vi "SaveScan_IM.vi"(10 "ScanSave Parameter":T1) -> (2 "Result":string)   [LabVIEW 2020]
panel:
  out "error out":errorcluster
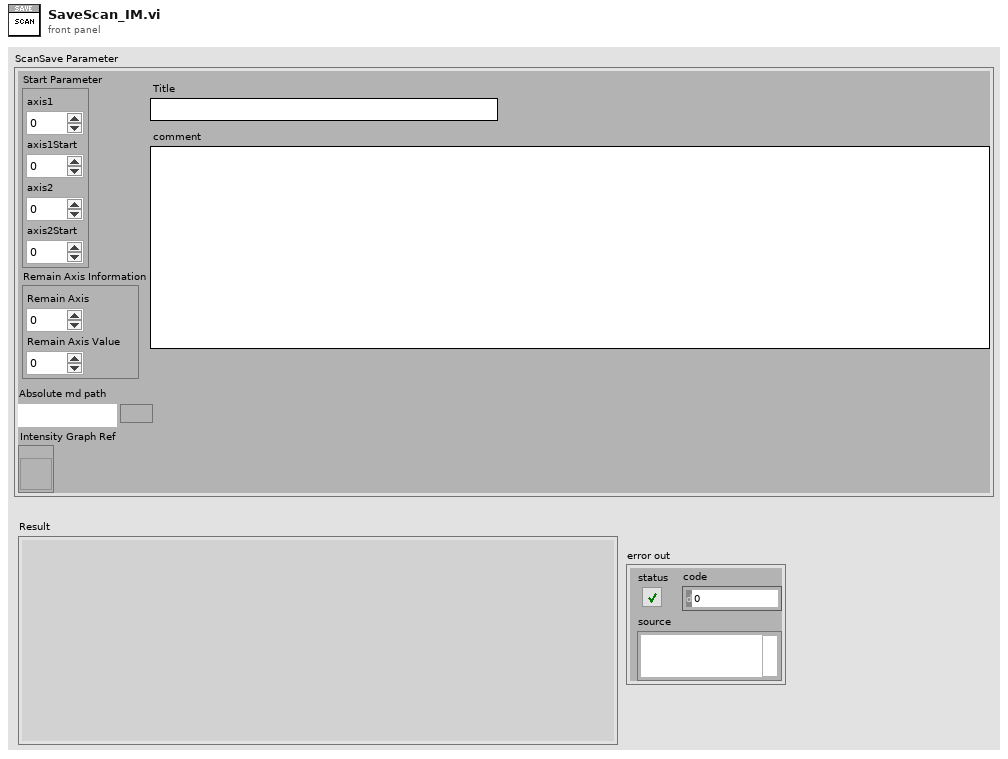
[diagram p1: front panel]
types:
  T1 = cluster{"Title":string, "Start Parameter":cluster{"axis1":i32, "axis1Start":dbl, "axis2":i32, "axis2Start":dbl}, "Remain Axis Information":cluster{"Remain Axis":i32, "Remain Axis Value":dbl}, "comment":string, "Absolute md path":path, "Intensity Graph Ref":refnum<vi>}
  T2 = enum16{"open", "replace", "create", "open or create", "replace or create", "replace or create with confirmation"}
  T3 = cluster{"axis1":i32, "axis1Start":dbl, "axis2":i32, "axis2Start":dbl}
  T4 = cluster{"Remain Axis":i32, "Remain Axis Value":dbl}
  T5 = enum32{"Bad", "Idle", "Run top level", "Running"}
  T6 = typedef "imagedata.ctl" = cluster{"image type":i32, "image depth":i32, "image":u8[], "mask":u8[], "colors":u32[], "Rectangle":cluster{"left":i16, "top":i16, "right":i16, "bottom":i16}}
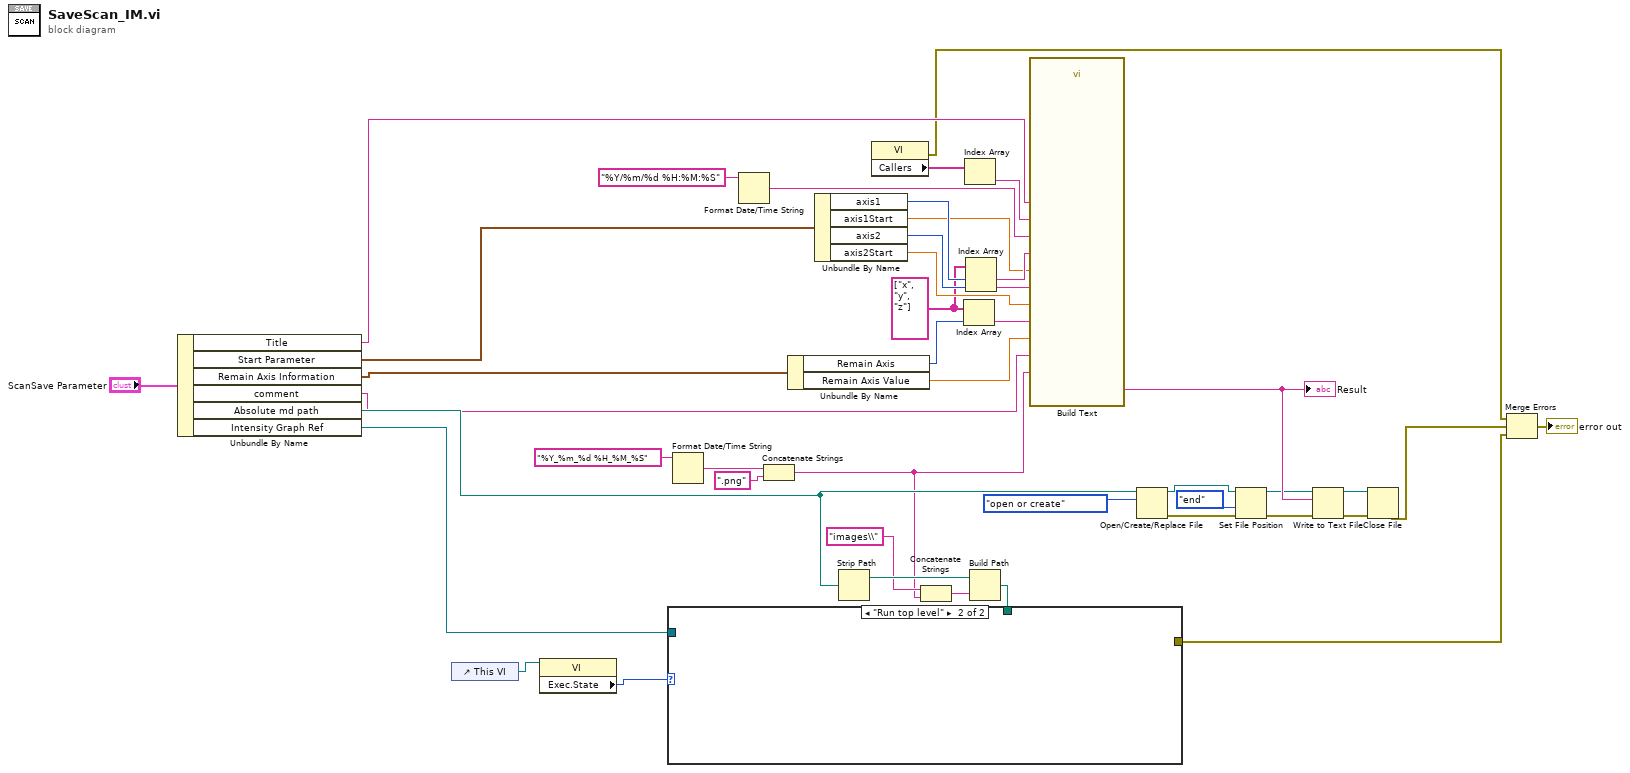
[diagram p0: block diagram]
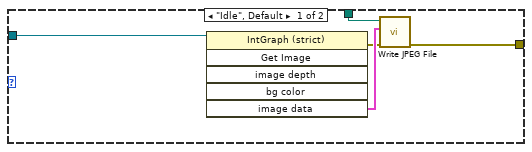
[diagram p2: hidden frame]
diagram:
  w33 = string[] ["x", "y", "z"]
  n1 = Unbundle By Name("ScanSave Parameter") -> ("Title"=w13:string, "Start Parameter"=w12:T3, "Remain Axis Information"=w11:T4, "comment"=w2:string, "Absolute md path"=w10:path, "Intensity Graph Ref"=w9:refnum<vi>)
  n2 = control-ref of="This VI"() -> (w23:refnum<vi>)
  n3 = property class="VI"(reference=w23) -> ("Exec.State"=w22:T5)  [unwired: 1 in, 2 out]
  n4 = Format Date/Time String(time format string (%c)="%Y_%m_%d %H_%M_%S") -> (date/time string=w3:string)  [unwired: 2 in]
  n5 = Format Date/Time String(time format string (%c)="%Y/%m/%d %H:%M:%S") -> (date/time string=w40:string)  [unwired: 2 in]
  n6 = Concatenate Strings(w3, ".png" ("string")) -> (w1:string)
  n7 = Unbundle By Name(w11) -> ("Remain Axis"=w32:i32, "Remain Axis Value"=w30:dbl)
  n8 = Unbundle By Name(w12) -> ("axis1"=w39:i32, "axis1Start"=w35:dbl, "axis2"=w38:i32, "axis2Start"=w34:dbl)
  n9 = Strip Path(path=w10) -> (stripped path=w29:path)  [unwired: 1 out]
  n10 = property class="VI"() -> (error out=w8:errorcluster, "Callers"=w43:string[])  [unwired: 2 in, 1 out]
  n11 = Concatenate Strings("images\\" ("string"), w1) -> (w16:string)
  n12 = Index Array(array=w33, index=w32) -> (element=w31:string)
  n13 = Index Array(array=w43) -> (element=w42:string)  [unwired: 1 in]
  n14 = Index Array(array=w33, index #1=w39, index #2=w38) -> (element #1=w37:string, element #2=w36:string)
  n15 = Build Path(base path=w29, name or relative path=w16) -> (appended path=w28:path)
  n16 = case shown="\"Run top level\"" w22 {
    tunnel: w28 -> [w49 _]
    tunnel: w9 -> [w46 _]
    tunnel: [w45 _] -> w6
    frame "Idle", Default {
      n17 = invoke class="IntGraph (strict)" method="Get Image"(reference=w46) -> (error out=w47:errorcluster, "image data"=w48:T6)  [unwired: 5 in, 4 out]
      n18 = call <vilib>:"Write JPEG File.vi"("error in (no error)"=w47, "image data"=w48, "path to JPEG file"=w49) -> ("error out"=w45:errorcluster)  [unwired: 8 out]
    }
    frame "Run top level" {
    }
  }
  n19 = call "Build Text"("Title"=w13, "VIname"=w42, "Time"=w40, "axis1"=w37, "axis1Start"=w35, "axis2"=w36, "axis2Start"=w34, "axis3"=w31, "axis3Start"=w30, "comment"=w2, "imgname"=w1) -> ("Result"=w25:string)  [unwired: 15 in, 1 out]
  "Result" <- w25
  n20 = Open/Create/Replace File(file path (use dialog)=w10, operation (0:open)=T2."open or create") -> (refnum out=w18:refnum<file>, error out=w20:errorcluster)  [unwired: 4 in, 1 out]
  n21 = Set File Position(refnum=w18, from (0:start)=enum16{"start", "end", "current"}."end", error in=w20) -> (refnum out=w17:refnum<file>, error out=w19:errorcluster)  [unwired: 1 in]
  n22 = Write to Text File(file (use dialog)=w17, text=w25, error in=w19) -> (refnum out=w26:refnum<file>, error out=w24:errorcluster)  [unwired: 1 in, 1 out]
  n23 = Close File(refnum=w26, error in=w24) -> (error out=w7:errorcluster)  [unwired: 1 out]
  n24 = Merge Errors(w8, w7, w6) -> (→"error out":errorcluster)
